vi "单按钮对话框示例.vi"   [LabVIEW 2021]
doc: "本VI是为《我和LabVIEW》一书编写的示例。\n关于本书的介绍请参考网页：\nhttp://ruanqizhen.spaces.live.com/blog/cns!5852D4F797C53FB6!4310.entry"
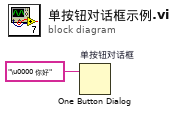
[diagram p0: block diagram]
diagram:
  n1 = One Button Dialog "单按钮对话框"(message="\u0000 你好") -> ()  [unwired: 2 out]
